vi "Open SHV Connections.vi"(8 "error in (no error)":errorcluster, 11 "Samples in":refnum<class "Samples.lvclass">) -> (0 "error out":errorcluster, 3 "Samples out":refnum<class "Samples.lvclass">)   [LabVIEW 2015, in "AMS UI.lvlib" / "Samples.lvclass"]
uses:
  Samples.lvclass
  Controls/Sample Line State Enumerator.ctl
  Samples.lvclass/Samples.ctl
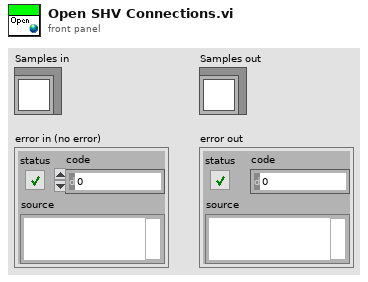
[diagram p1: front panel]
types:
  T1 = typedef "Sample Line State Enumerator.ctl" = enum16{"All lines closed", "Sample line 1.", "Sample line 2.", "Sample line 3.", "Sample line 4.", "Sample line 5.", "Out of range"}
  T2 = typedef "Sample Container.ctl" = cluster{"Sample In":refnum<k21>, "Sample Name":refnum<k21>, "Ti Cathode":refnum<k21>, "SampleQ":refnum<queue>}
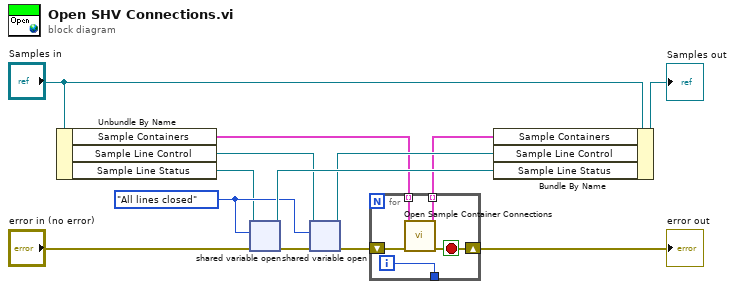
[diagram p0: block diagram]
diagram:
  w12 = Sample_Line_State_Enumerator."All lines closed" ("Enum")
  n1 = Unbundle By Name("Samples in") -> ("Sample Containers"=w3:T2[], "Sample Line Control"=w10:refnum<k21>, "Sample Line Status"=w7:refnum<k21>)
  n2 = shared-variable-open(w7, "error in (no error)", w12) -> (w13:refnum<k21>, w8:errorcluster)  [unwired: 1 in]
  n3 = shared-variable-open(w10, w8, w12) -> (w11:refnum<k21>, w4:errorcluster)  [unwired: 1 in]
  n4 = for {
    tunnel: w3 -> [w17] mode=indexing
    tunnel: [w16] -> w2 mode=indexing
    shift-right: [w15] -> w1
    shift-left: w4 -> [w18]
    tunnel: [w14] -> _
    i -> [w14]
    stop <- w15 stop-if-true
    n5 = call "Open Sample Container Connections.vi"("error in (no error)"=w18, "Container in"=w17) -> ("error out"=w15:errorcluster, "Container out"=w16:T2)  [unwired: 8 in]
  }
  "error out" <- w1
  n6 = Bundle By Name(cluster="Samples in", "Sample Containers"=w2, "Sample Line Control"=w11, "Sample Line Status"=w13) -> (→"Samples out":refnum<class "Samples.lvclass">)
